vi "Fix Streaming Data.vi"(8 "error in (no error)":errorcluster, 10 "ICM File In":path, 11 "Data String":string) -> (0 "error out":errorcluster, 3 "path":path)   [LabVIEW 2018]
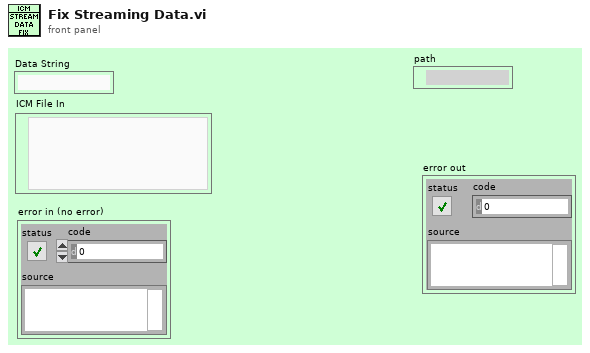
[diagram p1: front panel]
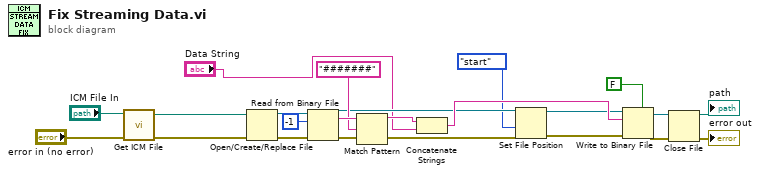
[diagram p0: block diagram]
diagram:
  n1 = call "Get ICM File.vi"("error in (no error)"="error in (no error)", "ICM File In"="ICM File In") -> ("error out"=w7:errorcluster, "ICM File"=w21:path)  [unwired: 8 in]
  n2 = Open/Create/Replace File(file path (use dialog)=w21, error in=w7) -> (refnum out=w20:refnum<file>, error out=w22:errorcluster)  [unwired: 4 in, 1 out]
  n3 = Read from Binary File(8:w22, 10:-1 ("count (1)"), 11:w20) -> (0:w10:errorcluster, 2:w19:string, 3:w12:refnum<file>)  [unwired: 3 in, 1 out]
  n4 = Match Pattern(string=w19, regular expression="#######") -> (before substring=w17:string)  [unwired: 1 in, 3 out]
  n5 = Concatenate Strings(w17, "Data String") -> (w16:string)
  n6 = Set File Position(refnum=w12, from (0:start)=enum16{"start", "end", "current"}."start", error in=w10) -> (refnum out=w11:refnum<file>, error out=w9:errorcluster)  [unwired: 1 in]
  n7 = Write to Binary File(file (use dialog)=w11, data=w16, error in=w9, 5:FALSE ("prepend array or string size? (T)")) -> (refnum out=w14:refnum<file>, error out=w15:errorcluster)  [unwired: 2 in, 1 out]
  n8 = Close File(refnum=w14, error in=w15) -> (path=→"path":path, error out=→"error out":errorcluster)
